vi "Write Hardware Settings.vi"(8 "error in (no error)":errorcluster, 10 "Hardware Settings.lvclass":refnum<class "Hardware Settings.lvclass">, 11 "Process Settings in":refnum<class "Process Settings.lvclass">) -> (0 "error out":errorcluster, 3 "Process Settings out":refnum<class "Process Settings.lvclass">)   [LabVIEW 2017, in "Process Settings.lvclass"]
uses:
  Process Settings.lvclass
  Hardware Settings/Hardware Settings.lvclass
  Process Settings.lvclass/Process Settings.ctl
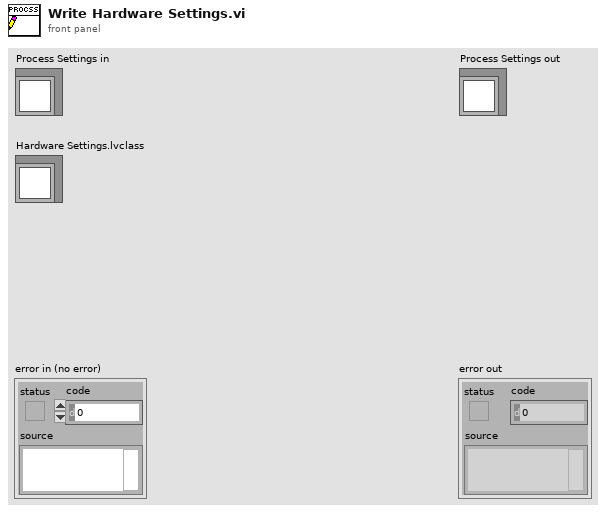
[diagram p1: front panel]
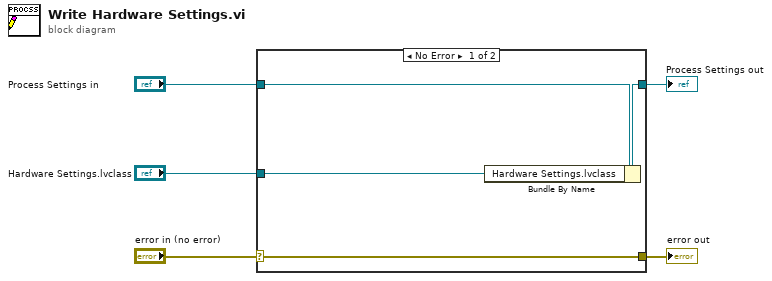
[diagram p0: block diagram]
diagram:
  n1 = case shown="No Error" "error in (no error)" {
    selector: "error in (no error)" -> [w9 w10]
    tunnel: [w9 w10] -> w4
    tunnel: [w7 w11] -> w2
    tunnel: "Process Settings in" -> [w8 w11]
    tunnel: "Hardware Settings.lvclass" -> [w6 _]
    frame No Error {
      n2 = Bundle By Name(cluster=w8, "Hardware Settings.lvclass"=w6) -> (w7:refnum<class "Process Settings.lvclass">)
    }
    frame Error {
    }
  }
  "error out" <- w4
  "Process Settings out" <- w2
